vi "CE14. parameter Read (SubVI).vi"(8 "error in (no error)":errorcluster, 11 "VISA Refnum in":refnum<visa-resource-name>) -> (0 "error out":errorcluster, 1 "dataout":T1, 2 "read buffer":string, 3 "VISA Refnum out":refnum<visa-resource-name>, 4 "time out":i32)   [LabVIEW 2018, in "CE14_eMIC.lvlib"]
uses:
  CE14_eMIC.lvlib
  type defs/CE14.data.ctl
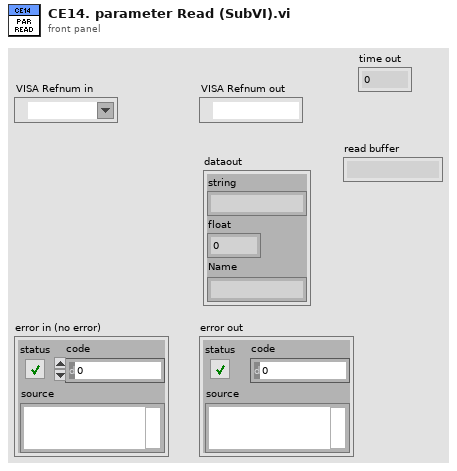
[diagram p1: front panel]
types:
  T1 = typedef "CE14_eMIC.lvlib/CE14.data.ctl" = cluster{"string":string, "float":dbl, "Name":string}
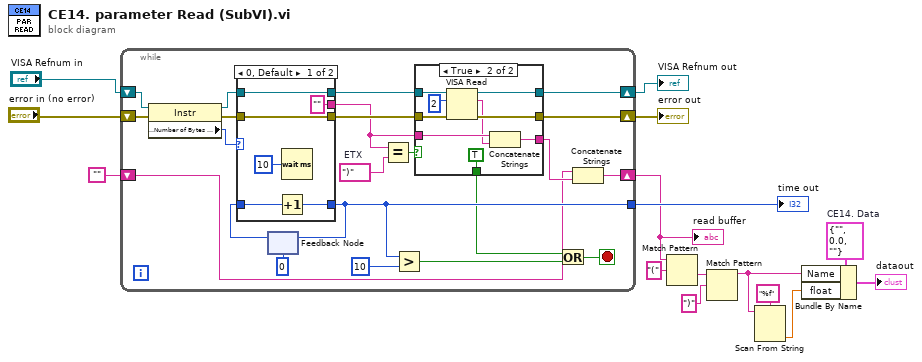
[diagram p0: block diagram]
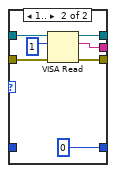
[diagram p2: hidden frame]
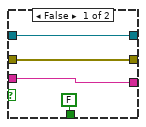
[diagram p3: hidden frame]
diagram:
  w12 = T1 {"string"="", "float"=0.0, "Name"=""}  # CE14. Data
  n1 = while {
    shift-right: [w27] -> w8
    shift-left: "error in (no error)" -> [w37]
    shift-right: [w26] -> w7
    shift-left: "VISA Refnum in" -> [w36]
    tunnel: [w21] -> w3
    shift-right: [w16] -> w1
    shift-left: "" -> [w17]
    stop <- w28 stop-if-true
    w23 = ")"  # ETX
    n2 = property class="Instr"(reference=w36, error in=w37) -> (reference out=w34:refnum<visa-resource-name>, error out=w35:errorcluster, "Serial Settings:Number of Bytes at Serial Port"=w33:u32)
    n3 = feedback #1(0) -> (w22:i32)
    n4 = case shown="0, Default" w33 {
      tunnel: w35 -> [w38 w50]
      tunnel: w34 -> [w43 w49]
      tunnel: [w43 w48] -> w30
      tunnel: [w38 w47] -> w29
      tunnel: ["" ("read buffer") w46] -> w24
      tunnel: w22 -> [w41 _]
      tunnel: [w40 0] -> w21
      frame 0, Default {
        n5 = Increment(x=w41) -> (x+1=w40:i32)
        n6 = Wait (ms)(milliseconds to wait=u32 10) -> ()  [unwired: 1 out]
      }
      frame 1.. {
        n7 = VISA Read(VISA resource name=w49, byte count=u32 1, error in (no error)=w50) -> (VISA resource name out=w48:refnum<visa-resource-name>, read buffer=w46:string, error out=w47:errorcluster)  [unwired: 1 out]
      }
    }
    n8 = feedback-in #1(w21) -> ()
    n9 = Equal?(x=w24, y=w23) -> (x = y?=w31:bool)
    n10 = Greater?(x=w21, y=10) -> (0:w19:bool)
    n11 = case shown="True" w31 {
      tunnel: w30 -> [w53 w63]
      tunnel: w29 -> [w52 w61]
      tunnel: [w52 w60] -> w27
      tunnel: [w53 w59] -> w26
      tunnel: [w54 w56] -> w25
      tunnel: w24 -> [w54 w58]
      tunnel: [FALSE TRUE] -> w18
      frame False {
      }
      frame True {
        n12 = VISA Read(VISA resource name=w63, byte count=u32 2, error in (no error)=w61) -> (VISA resource name out=w59:refnum<visa-resource-name>, read buffer=w57:string, error out=w60:errorcluster)  [unwired: 1 out]
        n13 = Concatenate Strings(w58, w57) -> (w56:string)
      }
    }
    n14 = Or(x=w18, y=w19) -> (x .or. y?=w28:bool)
    n15 = Concatenate Strings(w17, w25) -> (w16:string)
  }
  "VISA Refnum out" <- w7
  "error out" <- w8
  "read buffer" <- w1
  "time out" <- w3
  n16 = Match Pattern(string=w1, regular expression="(") -> (after substring=w10:string)  [unwired: 1 in, 3 out]
  n17 = Match Pattern(string=w10, regular expression=")") -> (before substring=w13:string)  [unwired: 1 in, 3 out]
  n18 = Scan From String(format string="%f", input string=w13) -> (output 1=w14:dbl)  [unwired: 3 in, 3 out]
  n19 = Bundle By Name(cluster=w12, "Name"=w13, "float"=w14) -> (→"dataout":T1)
